vi "process data buffer.vi"(5 "enabled":bool, 6 "completed packet queue":refnum<queue>, 7 "decimation":i32, 9 "nominal state":T1, 10 "Values":dbl[](array[numeric]), 11 "channel data in":T3) -> (2 "lost buffers":i32, 3 "channel data out":T3)   [LabVIEW 2026, in "Nominal Core Streaming Engine.lvlib"]
uses:
  Nominal Core Streaming Engine.lvlib
  rt full channel buffer.ctl
  rt per channel buffer.ctl
  nominal runtime state.ctl
  Shared/time convert type.ctl
  Shared/Nominal Core Streaming Shared.lvlib
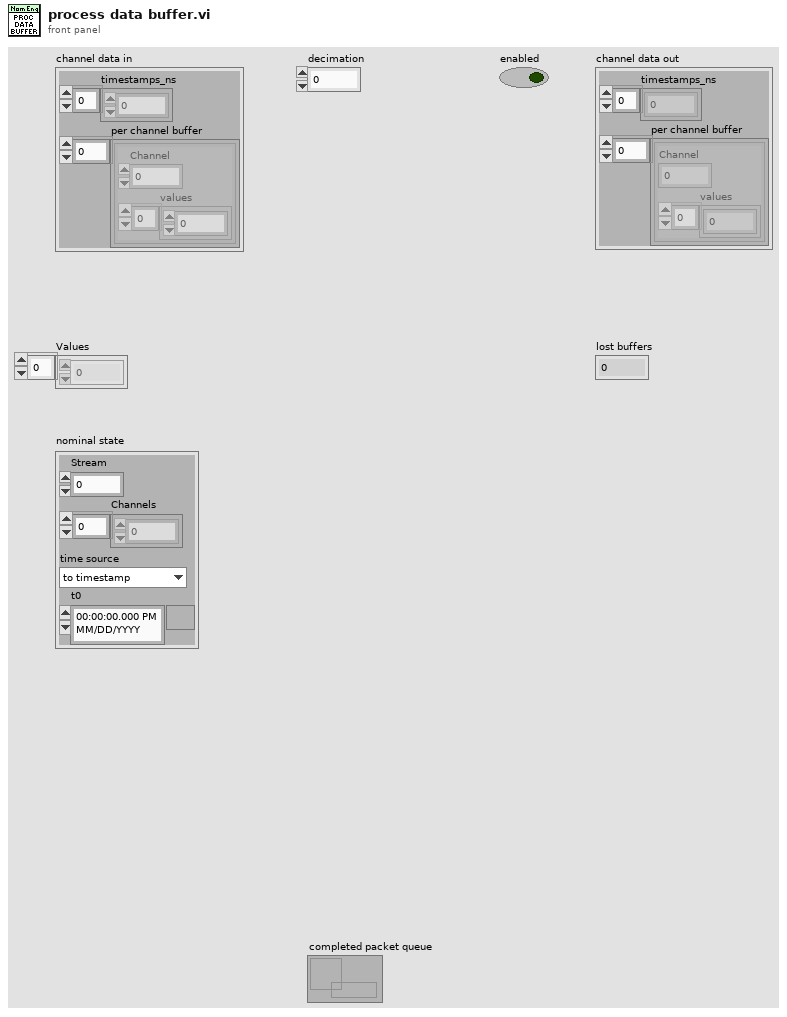
[diagram p1: front panel]
types:
  T1 = typedef "Nominal Core Streaming Engine.lvlib/nominal runtime state.ctl" = cluster{"Stream":u64, "Channels":u64[], "time source":T2, "t0":timestamp}
  T2 = typedef "Nominal Core Streaming Shared.lvlib/time convert type.ctl" = enum16{"to timestamp", "relative seconds"}
  T3 = typedef "Nominal Core Streaming Engine.lvlib/rt full channel buffer.ctl" = cluster{"timestamps_ns":i64[], "per channel buffer":T4[]}
  T4 = typedef "Nominal Core Streaming Engine.lvlib/rt per channel buffer.ctl" = cluster{"Channel":u64, "values":dbl[]}
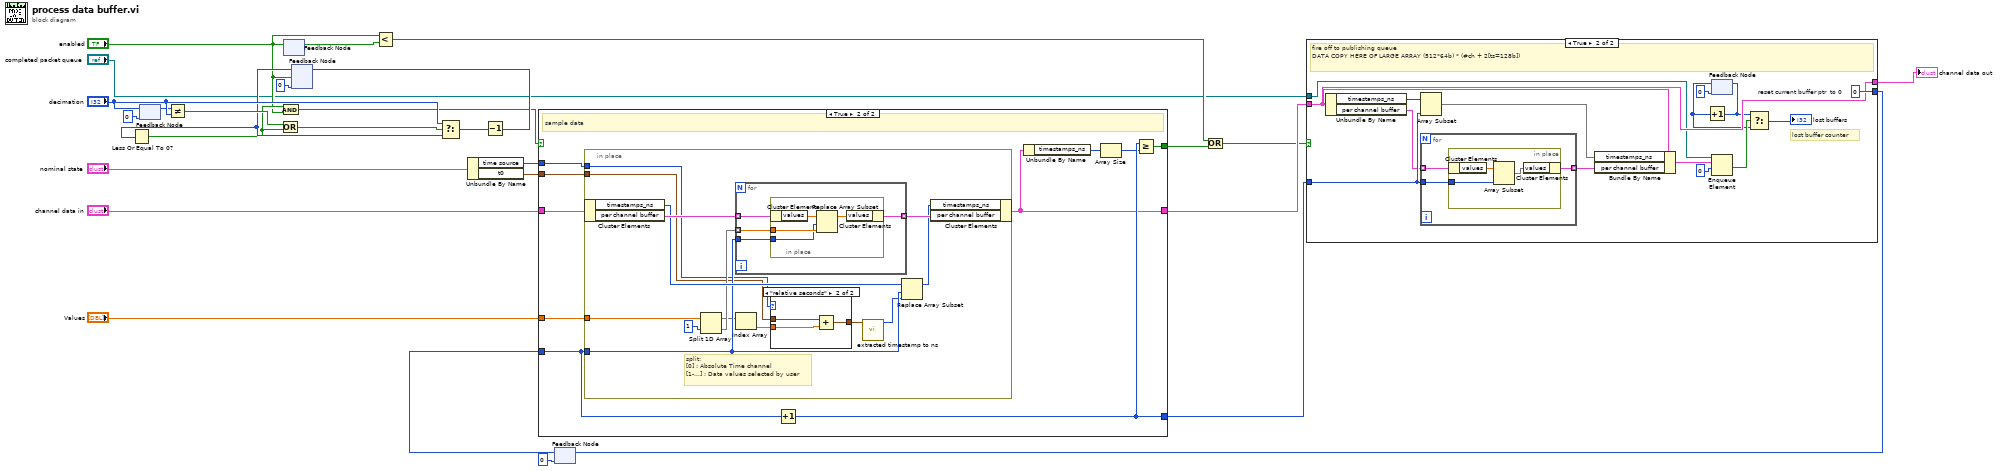
[diagram p0: block diagram]
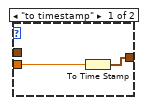
[diagram p3: hidden frame]
diagram:
  n1 = feedback #1(0 ("decimation")) -> (w26:i32)
  n2 = feedback-in #1("decimation") -> ()
  n3 = Not Equal?(x="decimation", y=w26) -> (x != y?=w25:bool)
  n4 = feedback #2() -> (w14:bool)  [unwired: 1 in]
  n5 = feedback-in #2("enabled") -> ()
  n6 = feedback #3(0) -> (w20:i32)
  n7 = Less Or Equal To 0?(x=w20) -> (x <= 0?=w19:bool)
  n8 = Or(x=w25, y=w19) -> (x .or. y?=w24:bool)
  n9 = And(x=w19, y="enabled") -> (x .and. y?=w13:bool)
  n10 = Less?(x="enabled", y=w14) -> (x < y?=w10:bool)
  n11 = Select(t="decimation", s=w24, f=w20) -> (s? t:f=w23:i32)
  n12 = Unbundle By Name("nominal state") -> ("time source"=w2:T2, "t0"=w1:timestamp)
  n13 = Decrement(x=w23) -> (x-1=w22:i32)
  n14 = feedback-in #3(w22, "enabled") -> ()
  n15 = feedback #4(0 ("decimation")) -> (w15:i32)
  n16 = case shown="True" w13 {
    tunnel: "channel data in" -> [w30 w36]
    tunnel: [w30 w33] -> w8
    tunnel: "Values" -> [_ w40]
    tunnel: w15 -> [w29 w39]
    tunnel: [w29 w38] -> w6
    tunnel: [_ w37] -> w11
    tunnel: w2 -> [_ w35]
    tunnel: w1 -> [_ w34]
    frame False {
      # "no sample for you"
    }
    frame True {
      # "sample data"
      n17 = in-place {
        in-place-border: w40 -> [w49]
        in-place-border: w39 -> [w51]
        in-place-border: w35 -> [w45]
        in-place-border: w34 -> [w44]
        # "split:\n[0] : Absolute Time channel\n[1-...] : Data values selected by user"
        n18 = in-place-cluster #5(w36) -> ("timestamps_ns"=w52:i64[], "per channel buffer"=w54:T4[])
        n19 = Split 1D Array(array=w49, index=1) -> (first subarray=w46:dbl[], second subarray=w47:dbl[])
        n20 = for {
          tunnel: w54 -> [w63] mode=indexing
          tunnel: [w62] -> w53 mode=indexing
          tunnel: w47 -> [w61] mode=indexing
          tunnel: w51 -> [w60]
          n21 = in-place {
            in-place-border: w61 -> [w66]
            in-place-border: w60 -> [w65]
            n22 = in-place-cluster #6(w63) -> ("values"=w67:dbl[])
            n23 = Replace Array Subset(array=w67, new element=w66, index=w65) -> (w64:dbl[])
            n24 = in-place-cluster #6("values"=w64) -> (w62:T4)
          }
        }
        n25 = Index Array(array=w46) -> (element=w43:dbl)  [unwired: 1 in]
        n26 = case shown="\"relative seconds\"" w45 {
          tunnel: w44 -> [_ w59]
          tunnel: w43 -> [w56 w58]
          tunnel: [w55 w57] -> w42
          frame "to timestamp" {
            n27 = To Time Stamp(1:w56) -> (0:w55:timestamp)
          }
          frame "relative seconds" {
            n28 = Add(x=w59, y=w58) -> (x+y=w57:timestamp)
          }
        }
        n29 = call "extracted timestamp to ns.vi"("Time Stamp"=w42) -> ("nominal core ns"=w41:i64)  [unwired: 10 in]
        n30 = Replace Array Subset(array=w52, new element=w41, index=w51) -> (w50:i64[])
        n31 = in-place-cluster #5("timestamps_ns"=w50, "per channel buffer"=w53) -> (w33:T3)
      }
      n32 = Increment(x=w39) -> (x+1=w38:i32)
      n33 = Unbundle By Name(w33) -> ("timestamps_ns"=w32:i64[])
      n34 = Array Size(array=w32) -> (size(s)=w31:i32)
      n35 = Greater Or Equal?(x=w38, y=w31) -> (x >= y?=w37:bool)
    }
  }
  n36 = Or(x=w10, y=w11) -> (x .or. y?=w7:bool)
  n37 = case shown="True" w7 {
    tunnel: [w69 w83] -> w9
    tunnel: w8 -> [w69 w83]
    tunnel: w6 -> [w68 w82]
    tunnel: [w68 w84] -> w5
    tunnel: "completed packet queue" -> [_ w77]
    frame False {
      # "keep on keepin on"
    }
    frame True {
      w84 = 0  # reset current buffer ptr  to 0
      # "lost buffer counter"
      # "fire off to publishing queue\nDATA COPY HERE OF LARGE ARRAY (512*64b) * (#ch + 2[ts=128b])"
      n38 = Unbundle By Name(w83) -> ("timestamps_ns"=w81:i64[], "per channel buffer"=w80:T4[])
      n39 = Array Subset(array=w81, length=w82) -> (w79:i64[])  [unwired: 1 in]
      n40 = for {
        tunnel: w82 -> [w87]
        tunnel: w80 -> [w86] mode=indexing
        tunnel: [w85] -> w78 mode=indexing
        n41 = in-place {
          in-place-border: w87 -> [w90]
          n42 = in-place-cluster #7(w86) -> ("values"=w89:dbl[])
          n43 = Array Subset(array=w89, length=w90) -> (w88:dbl[])  [unwired: 1 in]
          n44 = in-place-cluster #7("values"=w88) -> (w85:T4)
        }
      }
      n45 = Bundle By Name(cluster=w83, "timestamps_ns"=w79, "per channel buffer"=w78) -> (w76:T3)
      n46 = feedback #8(0 ("decimation")) -> (w71:i32)
      n47 = Increment(x=w71) -> (x+1=w72:i32)
      n48 = feedback-in #8(w72) -> ()
      n49 = Enqueue Element(queue=w77, element=w76, timeout in ms (-1)=0) -> (timed out?=w73:bool)  [unwired: 1 in, 2 out]
      n50 = Select(t=w72, s=w73, f=w71) -> (s? t:f=→"lost buffers":i32)
    }
  }
  "channel data out" <- w9
  n51 = feedback-in #4(w5) -> ()
